vi "Get - Vector - Complex.vi"(5 "use temporary file?":bool, 7 "data type of variable":cdb[](array[numeric]), 8 "error in":errorcluster, 10 "variable name":string, 11 "pipe in":T1) -> (0 "error out":errorcluster, 2 "value":cdb[](array[numeric]) format="%.2f", 3 "pipe out":T1)   [LabVIEW 2013, in "GOLPI library.lvlib"]
uses:
  GOLPI library.lvlib
  LV Process.lvlibp/Pipe Handle.ctl
  Custom Error Codes Enum Type Def.vi
  LV Process.lvlibp
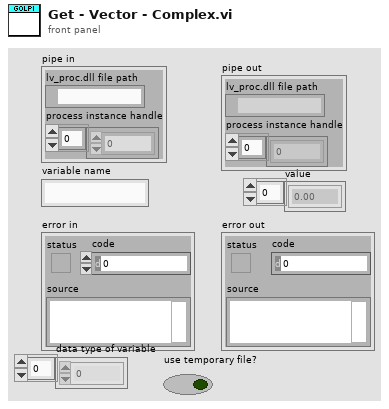
[diagram p1: front panel]
types:
  T1 = typedef "LV Process.lvlibp/Pipe Handle.ctl" = cluster{"lv_proc.dll file path":path, "process instance handle":u32[]}
  T2 = typedef "GOLPI library.lvlib/Custom Error Codes Enum Type Def.vi" = enum16{"no error", "00 working directory PAR1 missing", "01 octave binary PAR1 missing", "02 octave report error PAR1", "03 empty output last cmd PAR1", "04 missing temporary file PAR1", "10 var PAR1 not string", "11 var PAR1 not num, scal, ~compl", "12 var PAR1 not num, scal, compl", "13 var PAR1 not num, vect, ~compl", "14 var PAR1 not num, vect, compl", "15 var PAR1 not num, mat, ~compl", "16 var PAR1 not num, mat, ~compl", "99 not finished"}
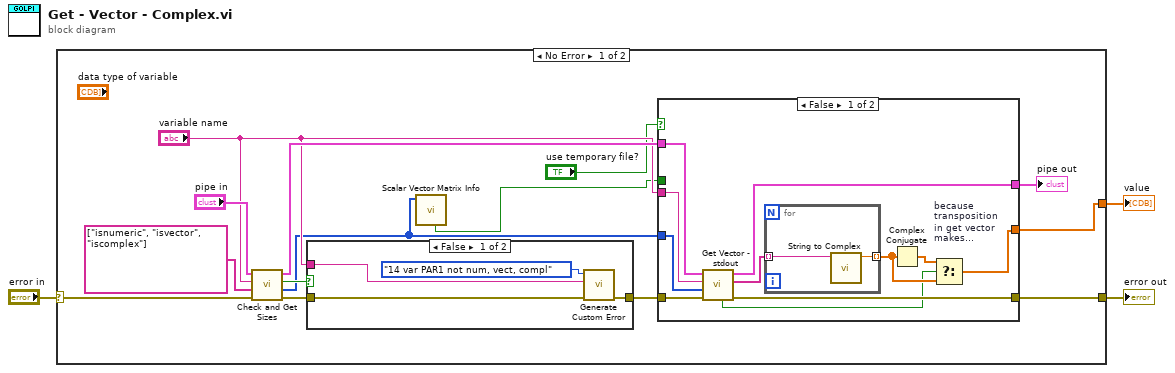
[diagram p0: block diagram]
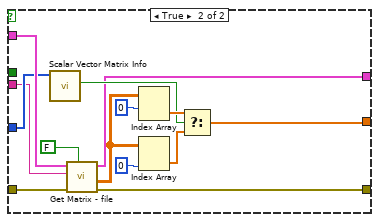
[diagram p2: hidden frame]
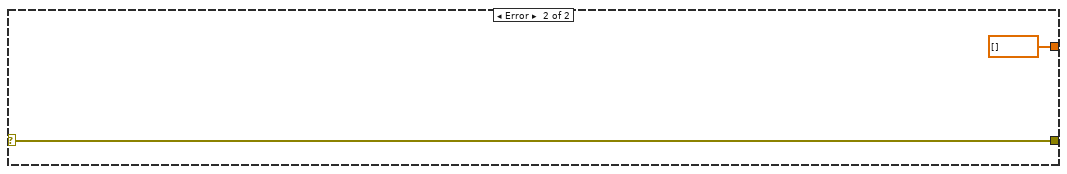
[diagram p4: hidden frame]
diagram:
  n1 = case shown="No Error" "error in" {
    selector: "error in" -> [w15 w51]
    tunnel: [w9 w51] -> w3
    tunnel: [w7 cdb[] [] ("value")] -> w1
    frame No Error {
      n2 = call "Check and Get Sizes.vi"("error in (no error)"=w15, "test commands"=string[] ["isnumeric", "isvector", "iscomplex"], "variable name"="variable name", "pipe in"="pipe in") -> ("error out"=w14:errorcluster, "octave sizes"=w5:i32[], "all tests OK?"=w16:bool, "pipe out"=w12:T1)  [unwired: 4 in]
      n3 = case shown="False" w16 {
        tunnel: w14 -> [w47 w49]
        tunnel: [w46 w49] -> w10
        tunnel: "variable name" -> [w45 _]
        frame False {
          n4 = call "Generate Custom Error.vi"("error in"=w47, "PAR1"=w45, "Enum"=Custom_Error_Codes_Enum_Type_Def.vi."14 var PAR1 not num, vect, compl") -> ("error out"=w46:errorcluster)  [unwired: 8 in]
        }
        frame True {
        }
      }
      n5 = call "Scalar Vector Matrix Info.vi"("octave sizes"=w5) -> ("row vector?"=w4:bool)  [unwired: 5 in, 5 out]
      n6 = case shown="False" "use temporary file?" {
        tunnel: w12 -> [w28 w35]
        tunnel: [w27 w36] -> w11
        tunnel: w10 -> [w26 w38]
        tunnel: [w25 w37] -> w9
        tunnel: w5 -> [w23 w32]
        tunnel: w4 -> [_ _]
        tunnel: "variable name" -> [w20 w31]
        tunnel: [w19 w33] -> w7
        frame False {
          n7 = call "Get Vector - stdout.vi"("error in (no error)"=w26, "octave vector sizes"=w23, "variable name"=w20, "pipe in"=w28) -> ("error out"=w25:errorcluster, "vector"=w24:string[], "pipe out"=w27:T1, "value transposed?"=w18:bool)  [unwired: 4 in]
          n8 = for {
            tunnel: w24 -> [w30] mode=indexing
            tunnel: [w29] -> w21 mode=indexing
            n9 = call "String to Complex.vi"("string"=w30) -> ("complex number"=w29:cdb)  [unwired: 10 in]
          }
          n10 = Complex Conjugate(1:w21) -> (0:w22:cdb[])
          n11 = Select "because\ntransposition\nin get vector\nmakes\nconjugate"(t=w22, s=w18, f=w21) -> (s? t:f=w19:cdb[])
        }
        frame True {
          n12 = call "Scalar Vector Matrix Info.vi"("octave sizes"=w32) -> ("is vector?"=w40:bool)  [unwired: 5 in, 5 out]
          n13 = call "Get Matrix - file.vi"("is string"=FALSE, "error in (no error)"=w38, "variable name"=w31, "pipe in"=w35) -> ("error out"=w37:errorcluster, "cmplx double array"=w34:cdb[][], "pipe out"=w36:T1)  [unwired: 3 in, 2 out]
          n14 = Index Array(array=w34, index (row)=0) -> (element=w42:cdb[])  [unwired: 1 in]
          n15 = Index Array(array=w34, index (col)=0 ("disabled index (col)")) -> (element=w41:cdb[])  [unwired: 1 in]
          n16 = Select(t=w42, s=w40, f=w41) -> (s? t:f=w33:cdb[])
        }
      }
      "pipe out" <- w11
    }
    frame Error {
    }
  }
  "value" <- w1
  "error out" <- w3
